vi "PrefToXMLItems.vi"(8 "error in (no error)":errorcluster, 11 "Preferences in":refnum<class "SetListPrefs.lvclass">) -> (0 "error out":errorcluster, 2 "XMLArray":string[](array[string]), 3 "Preferences out":refnum<class "SetListPrefs.lvclass">)   [LabVIEW 2013, in "SetListPrefs.lvclass"]
uses:
  SetListPrefs.lvclass
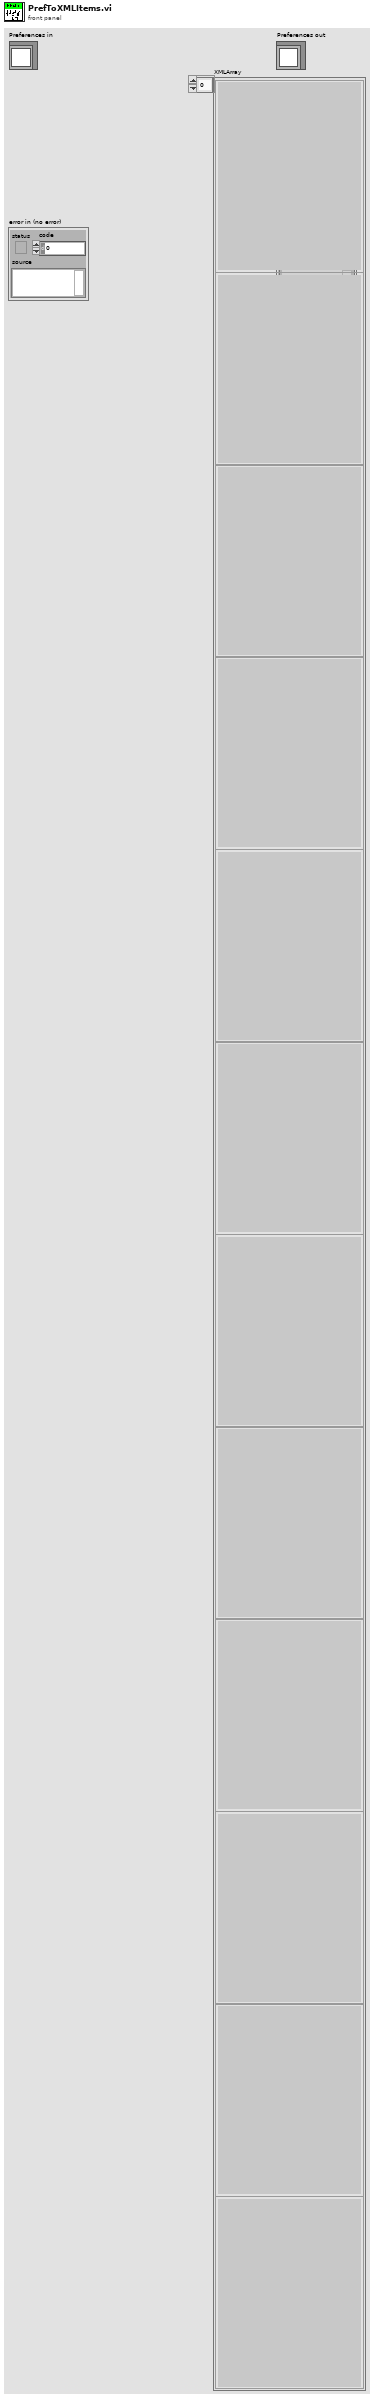
[diagram p1: front panel]
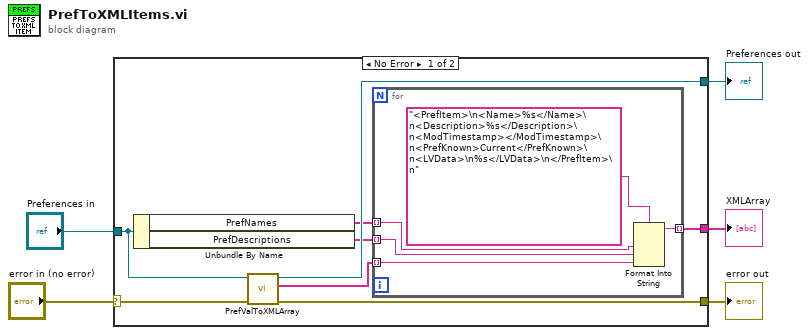
[diagram p0: block diagram]
diagram:
  n1 = case shown="No Error" "error in (no error)" {
    selector: "error in (no error)" -> [w11 w20]
    tunnel: [w10 w20] -> w4
    tunnel: [w12 w19] -> w2
    tunnel: "Preferences in" -> [w13 w19]
    tunnel: [w6 _] -> w1
    frame No Error {
      n2 = Unbundle By Name(w13) -> ("PrefNames"=w8:string[], "PrefDescriptions"=w9:string[])
      n3 = call "PrefValToXMLArray.vi"("error in (no error)"=w11, "Preferences in"=w13) -> ("error out"=w10:errorcluster, "PrefXML"=w7:string[], "Preferences out"=w12:refnum<class "SetListPrefs.lvclass">)  [unwired: 7 in]
      n4 = for {
        tunnel: w9 -> [w16] mode=indexing
        tunnel: w8 -> [w17] mode=indexing
        tunnel: w7 -> [w15] mode=indexing
        tunnel: [w14] -> w6 mode=indexing
        n5 = Format Into String(format string="<PrefItem>\n<Name>%s</Name>\n<Description>%s</Description>\n<ModTimestamp></ModTimestamp>\n<PrefKnown>Current</PrefKnown>\n<LVData>\n%s</LVData>\n</PrefItem>\n", w17, w16, w15) -> (resulting string=w14:string)  [unwired: 2 in, 1 out]
      }
    }
    frame Error {
    }
  }
  "error out" <- w4
  "Preferences out" <- w2
  "XMLArray" <- w1
